vi "rs3 stop 3.vi"(8 "error in (no error)":errorcluster, 11 "device":u64) -> (0 "error out":errorcluster, 2 "device out":u64)   [LabVIEW 2023]
doc: "Stops streaming on the specified sensor."
panel:
  # "RS3 Stop"
  # "(C) Intel Corp. 2017,  AGJ"
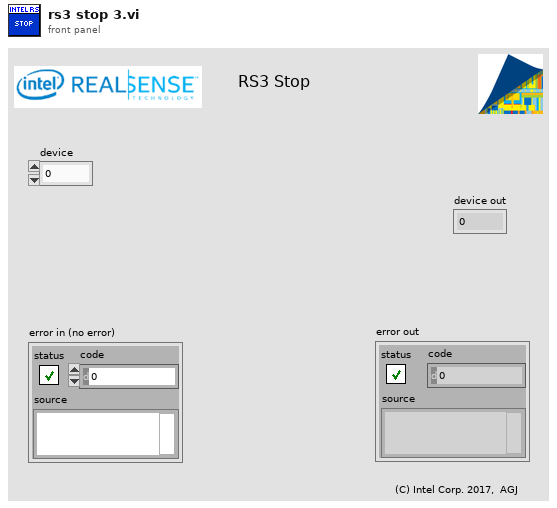
[diagram p1: front panel]
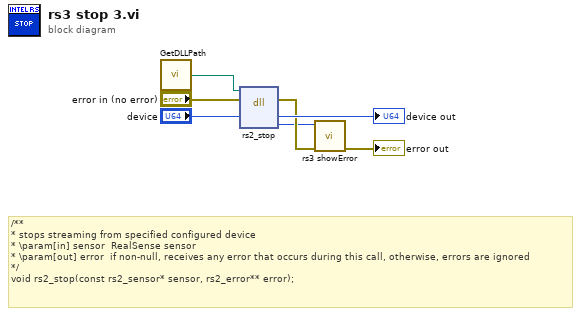
[diagram p0: block diagram]
diagram:
  # "/**\n* stops streaming from specified configured device\n* \\param[in] sensor  RealSense sensor\n* \\param[out] error  if non-null, receives any error that occurs during this call, otherwise, errors are ignored\n*/\nvoid rs2_stop(const rs2_sensor* sensor, rs2_error** error);"
  n1 = call "GetDLLPath.vi"() -> ("DLL Path"=w1:path)
  n2 = dll-call lib="C:/STEAMSyndicate/RealSenseWrappers/VI Wrappers (add ons) Public/RealSense/realsense2.dll" fn="rs2_stop"(path in=w1, error in="error in (no error)", "device"="device") -> (error out=w3:errorcluster, "device"=→"device out":u64, "error"=w2:u64)  [unwired: 3 in, 1 out]
  n3 = call "rs3 showError.vi"("error in (no error)"=w3, "error"=w2) -> ("error out"=→"error out":errorcluster)  [unwired: 5 in, 4 out]
